vi "Teleop.vi"(10 "Match Info":T2={"Autonomous Elapsed Seconds"=0.0, "TeleOp Elapsed Seconds"=0.0, "Disabled Elapsed Seconds"=0.0, "Visited Autonomous"=FALSE, "Visited TeleOp"=FALSE, "Visited Disabled"=FALSE, "Autonomous Settings"={"Autonomous Style"=enum."Independent", "VI Refnum"=refnum}}, 11 "Call Context":T3) -> ()   [LabVIEW 2015]
doc: "This VI is called for each TeleOp packet received from the DS where the robot is not disabled. It is often used to read from the joysticks and update I/O or to update setpoints for timed control loops. It should complete and return within 20 milliseconds or it may miss DS packets."
uses:
  <vilib>/Rock Robotics/WPI/DriverStation/WPI_DriverStationDerivedRobotMode.ctl
  <vilib>/Rock Robotics/WPI/DriverStation/WPI_DriverStationMatch Info.ctl
  <vilib>/Rock Robotics/WPI/CAN/TalonSRX/WPI_CANTalonSRX_GlobalStatus.ctl
  <vilib>/Rock Robotics/WPI/Utilities/WPI_GetSetVariantRefNum.vi
  <vilib>/Rock Robotics/Network Tables/NT Write Boolean Array.vi
  <vilib>/Rock Robotics/Network Tables/NT Write Numeric Array.vi
  <vilib>/Rock Robotics/Network Tables/NT Read Boolean.vi
  <vilib>/Rock Robotics/Network Tables/NT Read Number.vi
  Stage.vi
panel:
  out "Set Point":dbl
  out "Talon SRX Status":T1
  out "Waveform Chart":cluster{"Encoder Velocity":dbl, dbl}(graph)
  out "Encoder Velocity":dbl
  out "Mode":bool
  out "Pos":bool
  out "Arm":dbl
  out "Optic":bool
  out "B10":bool
  out "B9":bool
  out "B8":bool
  out "Shooter rpm":dbl
  out "hooks motor":dbl
  out "Winch":dbl
  out "Stage3Motor":dbl
  out "Drive":dbl=0.5
  out "Stage1Motor":dbl
  out "Stage":dbl
  out "B7":bool
  out "ALU":bool
  out "ALB":bool
  out "B6":bool
  out "B5":bool
  out "LT":bool
  out "LM":bool
  out "LB":bool
  out "B4":bool
  out "B3":bool
  out "B2":bool
  out "B1":bool
  out "B0":bool
  out "Full speed":bool=TRUE
  out "Sample Slider 0":dbl(slide) scale=0.0..5.0
  out "Sample Boolean 1":bool
  out "Sample Boolean 0":bool
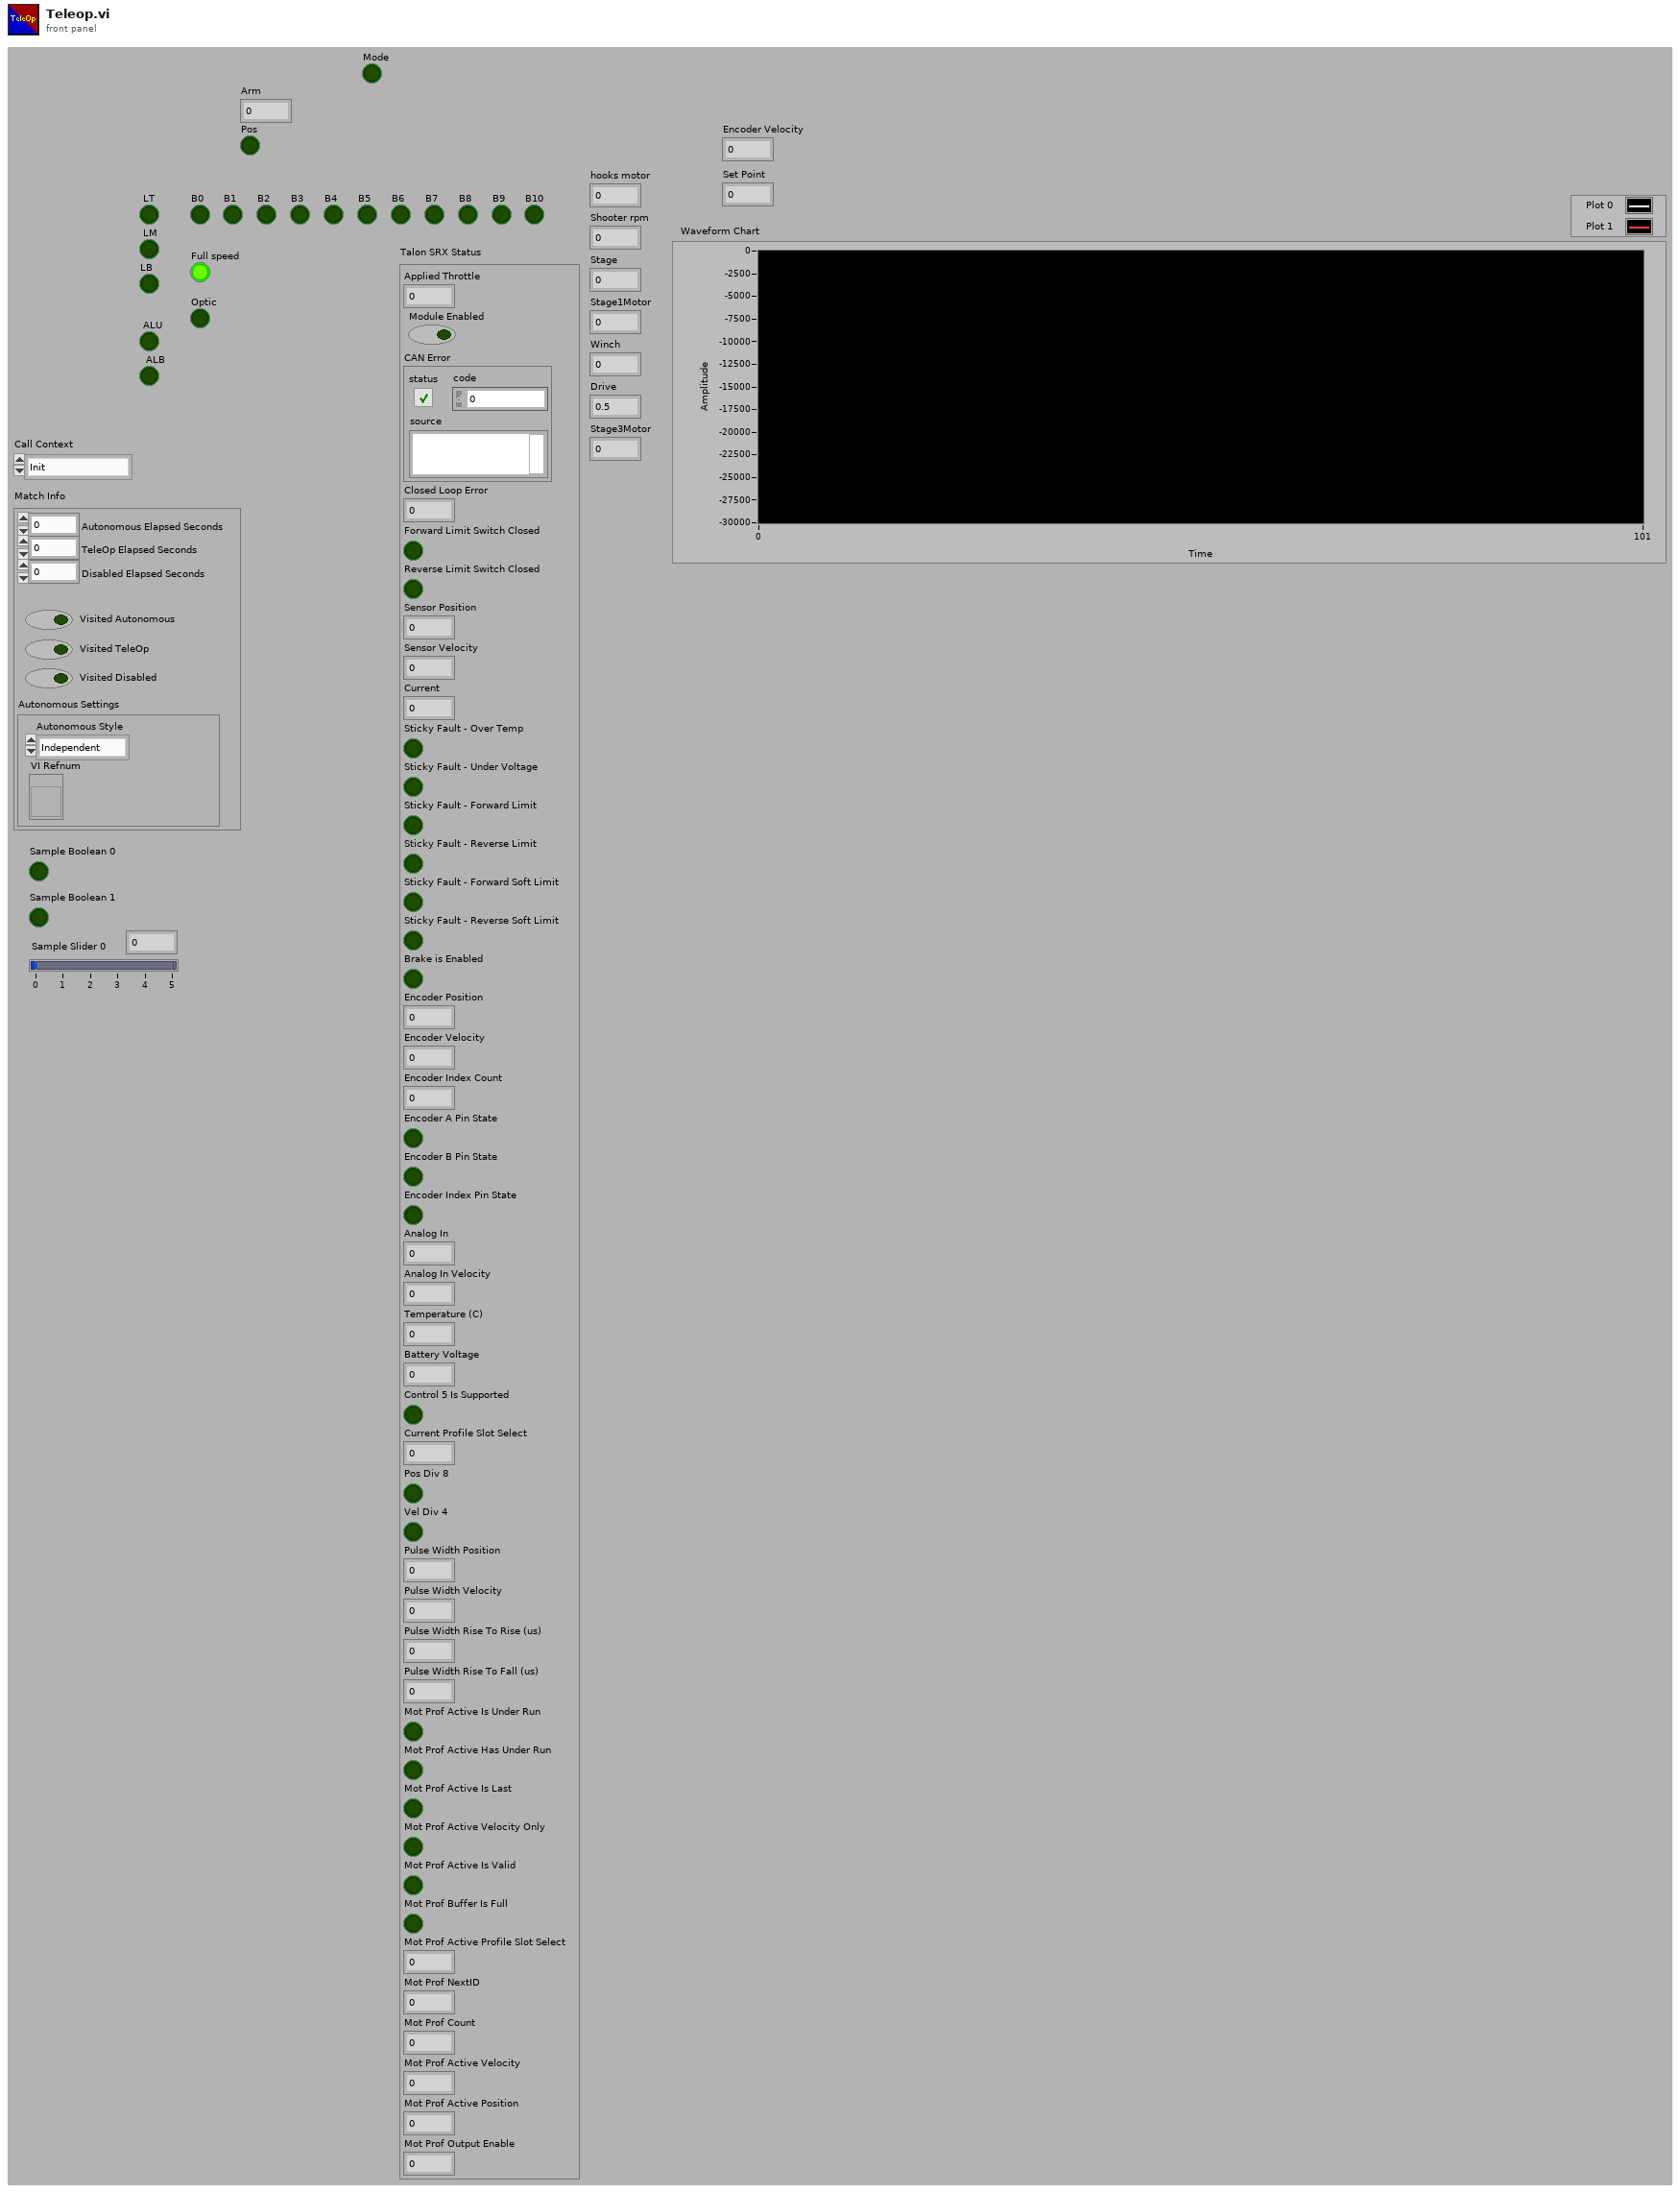
[diagram p1: front panel]
types:
  T1 = typedef "WPI_CANTalonSRX_GlobalStatus.ctl" = cluster{"Applied Throttle":dbl, "Module Enabled":bool, "CAN Error":errorcluster, "Closed Loop Error":dbl, "Forward Limit Switch Closed":bool, "Reverse Limit Switch Closed":bool, "Sensor Position":dbl, "Sensor Velocity":dbl, "Current":dbl, "Sticky Fault - Over Temp":bool, "Sticky Fault - Under Voltage":bool, "Sticky Fault - Forward Limit":bool, "Sticky Fault - Reverse Limit":bool, "Sticky Fault - Forward Soft Limit":bool, "Sticky Fault - Reverse Soft Limit":bool, "Brake is Enabled":bool, "Encoder Position":dbl, "Encoder Velocity":dbl, "Encoder Index Count":dbl, "Encoder A Pin State":bool, "Encoder B Pin State":bool, "Encoder Index Pin State":bool, "Analog In":dbl, "Analog In Velocity":dbl, "Temperature (C)":dbl, "Battery Voltage":dbl, "Control 5 Is Supported":bool, "Current Profile Slot Select":dbl, "Pos Div 8":bool, "Vel Div 4":bool, "Pulse Width Position":i32, "Pulse Width Velocity":i32, "Pulse Width Rise To Rise (us)":i32, "Pulse Width Rise To Fall (us)":i32, "Mot Prof Active Is Under Run":bool, "Mot Prof Active Has Under Run":bool, "Mot Prof Active Is Last":bool, "Mot Prof Active Velocity Only":bool, "Mot Prof Active Is Valid":bool, "Mot Prof Buffer Is Full":bool, "Mot Prof Active Profile Slot Select":i32, "Mot Prof NextID":i32, "Mot Prof Count":i32, "Mot Prof Active Velocity":dbl, "Mot Prof Active Position":dbl, "Mot Prof Output Enable":i32}
  T2 = typedef "WPI_DriverStationMatch Info.ctl" = cluster{"Autonomous Elapsed Seconds":dbl, "TeleOp Elapsed Seconds":dbl, "Disabled Elapsed Seconds":dbl, "Visited Autonomous":bool, "Visited TeleOp":bool, "Visited Disabled":bool, "Autonomous Settings":cluster{"Autonomous Style":enum16{"Iterative", "Independent"}, "VI Refnum":refnum<vi>}}
  T3 = typedef "WPI_DriverStationDerivedRobotMode.ctl" = enum16{"Init", "Execute", "Stop"}
  T4 = typedef "WPI_DigitalInputDevRef.ctl" = cluster{"DevStatus":errorcluster, "DIO Channel":T5}
  T5 = typedef "FPGA_DIOChannel.ctl" = enum8{"DIO 0", "DIO 1", "DIO 2", "DIO 3", "DIO 4", "DIO 5", "DIO 6", "DIO 7", "DIO 8", "DIO 9", "DIO MXP 0", "DIO MXP 1", "DIO MXP 2", "DIO MXP 3", "DIO MXP 4", "DIO MXP 5", "DIO MXP 6", "DIO MXP 7", "DIO MXP 8", "DIO MXP 9", "DIO MXP 10", "DIO MXP 11", "DIO MXP 12", "DIO MXP 13", "DIO MXP 14", "DIO MXP 15", "Invalid"}
  T6 = typedef "WPI_RobotDriveDevRef.ctl" = cluster{"DevStatus":errorcluster, "Motors[]":T7[], "Square Inputs":bool, "Max Output":dbl}
  T7 = typedef "WPI_MotorControlDeviceRef.ctl" = cluster{"DeviceStatus":errorcluster, "Type":T8, "PWM":cluster{"PWM Channel":T9, "DeadBand":T10}, "CAN":cluster{"Device Number":u8, "Control Mode":T11, "Semaphore":T12, "Max Vout":dbl, "TalonSRX Control Mode":T13}, "Invert":bool}
  T8 = typedef "WPI_MotorControlType.ctl" = enum16{"PWM", "CAN", "CANTalonSRX"}
  T9 = typedef "FPGA_DIOPWMChannel.ctl" = enum8{"PWM 0", "PWM 1", "PWM 2", "PWM 3", "PWM 4", "PWM 5", "PWM 6", "PWM 7", "PWM 8", "PWM 9", "PWM MXP 0", "PWM MXP 1", "PWM MXP 2", "PWM MXP 3", "PWM MXP 4", "PWM MXP 5", "PWM MXP 6", "PWM MXP 7", "PWM MXP 8", "PWM MXP 9", "Invalid"}
  T10 = typedef "WPI_PWMDeadband.ctl" = cluster{"Name":string, "maxPositivePwm":i32, "minPositivePwm":i32, "centerPwm":i32, "maxNegativePwm":i32, "minNegativePwm":i32, "angularRange":u16}
  T11 = typedef "WPI_CANJaguar_ControlMode.ctl" = enum8{"Percent VBus", "Current", "Speed", "Position", "Voltage"}
  T12 = typedef "Semaphore RefNum" = refnum<k1>
  T13 = typedef "WPI_CANTalonSRX_APIControlMode.ctl" = enum8{"Percent VBus", "Speed", "Position", "Slave", "Unchanged / Invalid", "Voltage Compensation", "Current", "Motion Profile"}
  T14 = typedef "WPI_JoystickDevRef.ctl" = cluster{"Device":T15}
  T15 = typedef "WPI_JoystickDeviceEnum.ctl" = enum16{"USB 0", "USB 1", "USB 2", "USB 3", "USB 4", "USB 5"}
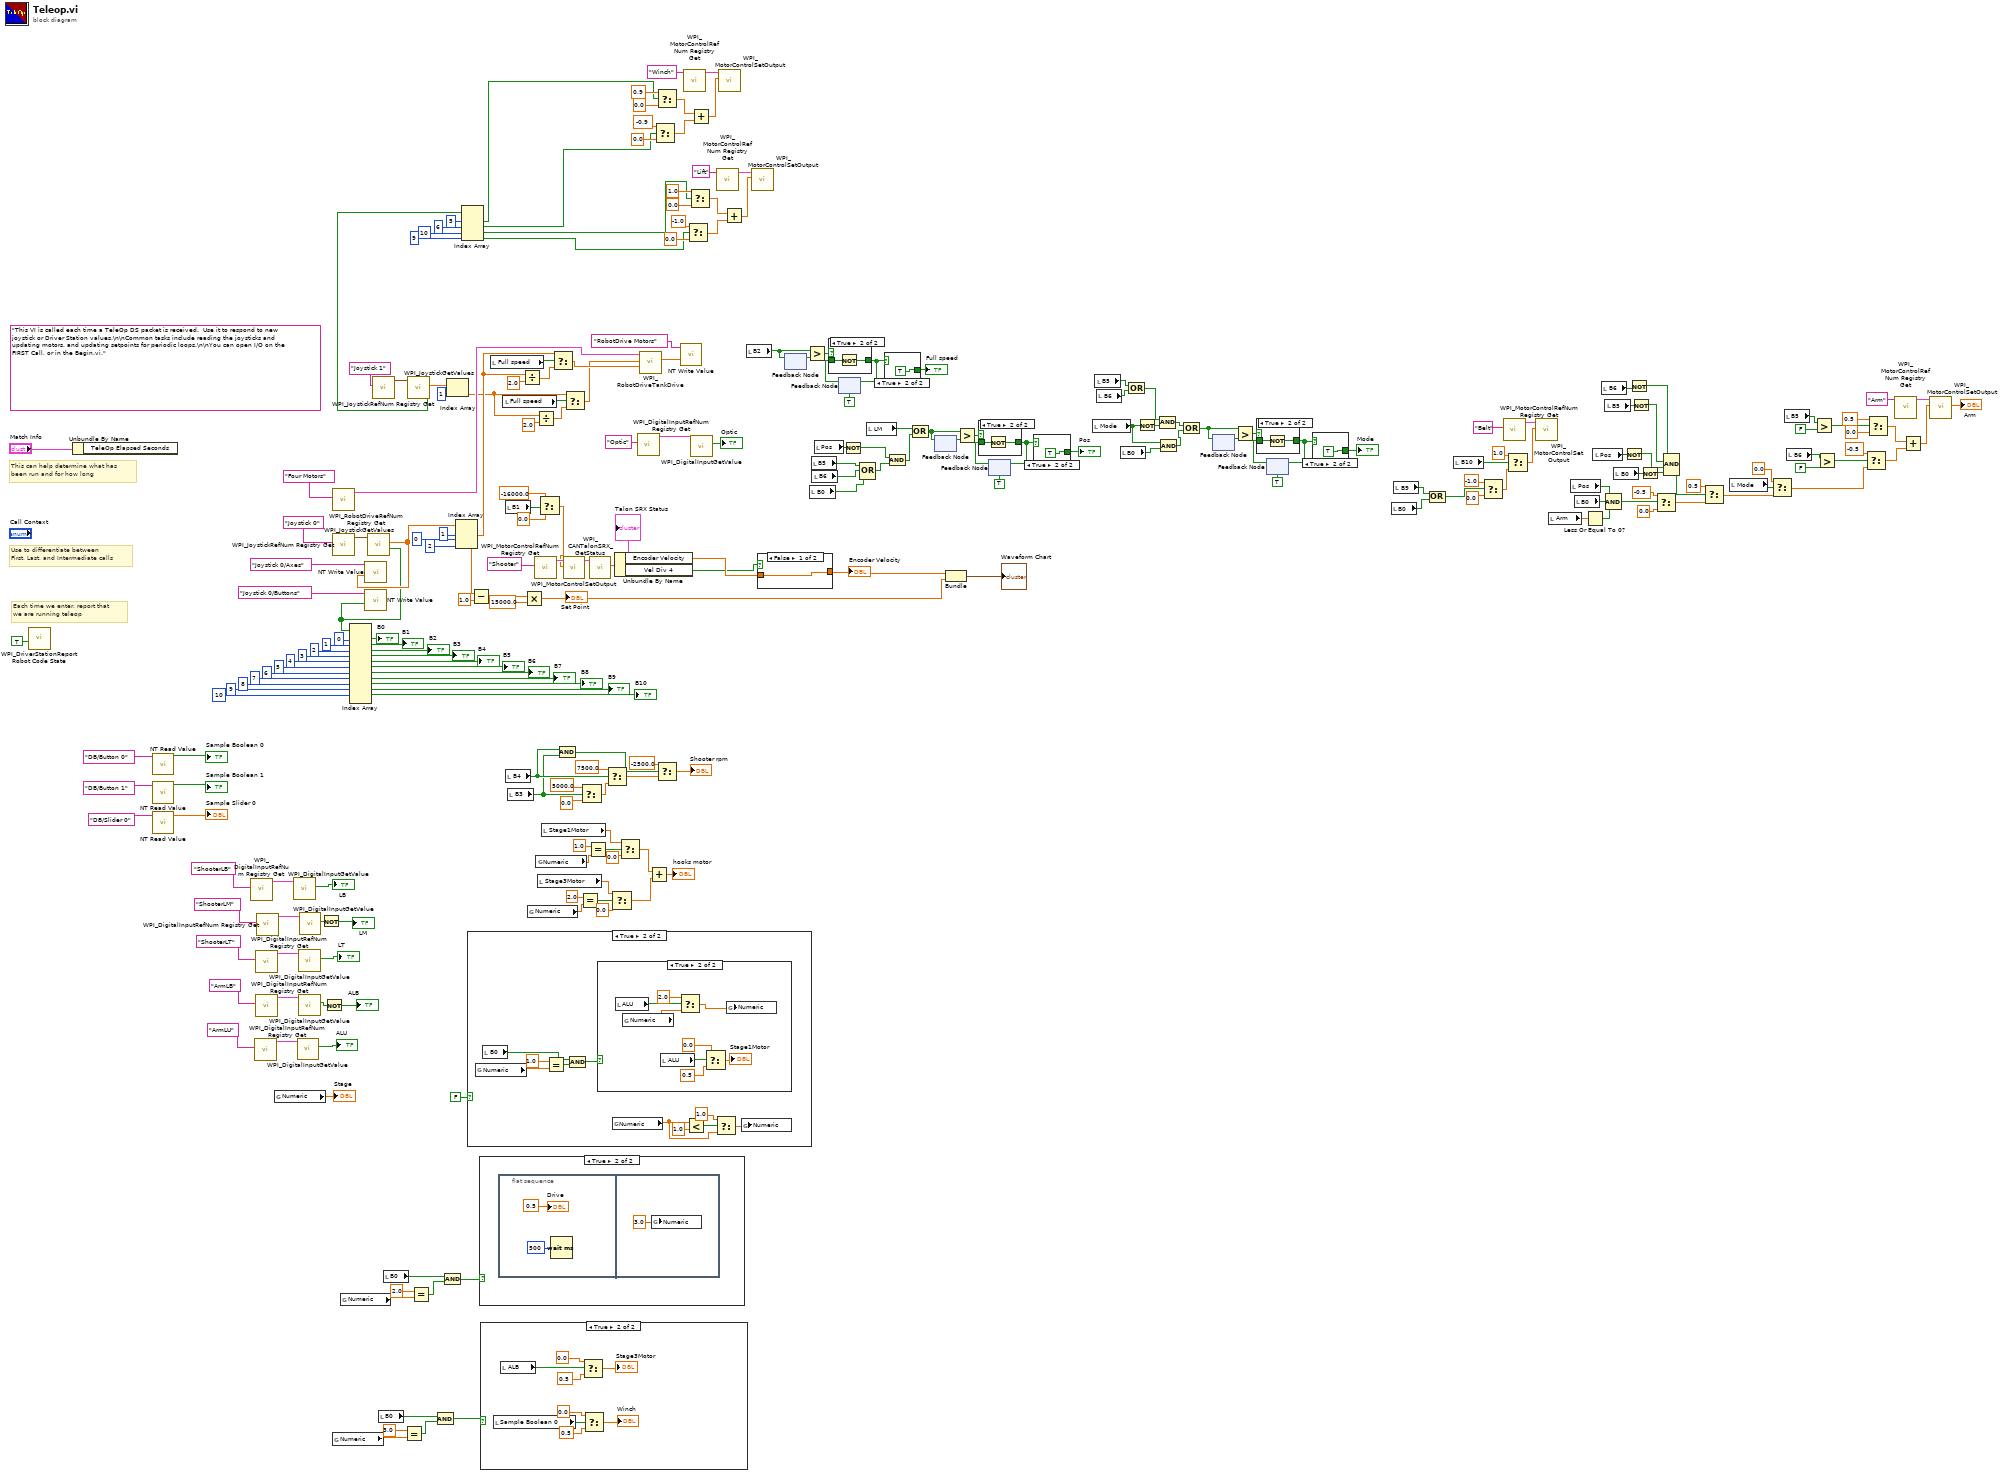
[diagram p0: block diagram]
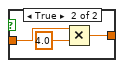
[diagram p2: hidden frame]
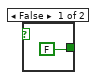
[diagram p3: hidden frame]
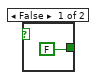
[diagram p5: hidden frame]
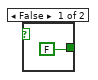
[diagram p11: hidden frame]
diagram:
  (unwired) "This VI is called each time a TeleOp DS packet is received.  Use it to respond to new joystick or Driver Station values.\n\nCommon tasks include reading the joysticks and updating motors, and updating setpoints for periodic loops.\n\nYou can open I/O on the FIRST Call, or in the Begin.vi."
  # "Each time we enter, report that\nwe are running teleop"
  # "Use to differentiate between\nFirst, Last, and Intermediate calls"
  # "This can help determine what has\nbeen run and for how long"
  n1 = call <vilib>:"WPI_DriverStationReport Robot Code State.vi"("TeleOp"=TRUE ("Autonomous")) -> ()  [unwired: 10 in, 1 out]
  n2 = Unbundle By Name("Match Info") -> ()  [unwired: 1 out]
  n3 = call-poly <vilib>:"NT Read Value.vi"("Name"="DB/Button 0" ("refnum name")) -> ("Boolean"=→"Sample Boolean 0":bool)  [unwired: 9 in, 1 out]
  n4 = call-poly <vilib>:"NT Read Value.vi"("Name"="DB/Button 1" ("refnum name")) -> ("Boolean"=→"Sample Boolean 1":bool)  [unwired: 9 in, 1 out]
  n5 = call-poly <vilib>:"NT Read Value.vi"("Name"="DB/Slider 0" ("refnum name")) -> ("Numeric"=→"Sample Slider 0":dbl)  [unwired: 9 in, 1 out]
  n6 = call <vilib>:"WPI_DigitalInputRefNum Registry Get.vi"("refnum name"="ShooterLB") -> ("DigitalInputDevRef"=w188:T4)  [unwired: 9 in, 1 out]
  n7 = call <vilib>:"WPI_DigitalInputRefNum Registry Get.vi"("refnum name"="ArmLU") -> ("DigitalInputDevRef"=w163:T4)  [unwired: 9 in, 1 out]
  n8 = call <vilib>:"WPI_DigitalInputRefNum Registry Get.vi"("refnum name"="ShooterLT") -> ("DigitalInputDevRef"=w183:T4)  [unwired: 9 in, 1 out]
  n9 = call <vilib>:"WPI_DigitalInputRefNum Registry Get.vi"("refnum name"="ArmLB") -> ("DigitalInputDevRef"=w164:T4)  [unwired: 9 in, 1 out]
  n10 = call <vilib>:"WPI_DigitalInputRefNum Registry Get.vi"("refnum name"="ShooterLM") -> ("DigitalInputDevRef"=w184:T4)  [unwired: 9 in, 1 out]
  n11 = global read "Stage.vi" "Numeric"() -> (→"Stage":dbl)
  n12 = call <vilib>:"WPI_DigitalInputGetValue.vi"("DigitalInputDevRef"=w188) -> ("Value"=→"LB":bool)  [unwired: 8 in, 2 out]
  n13 = call <vilib>:"WPI_DigitalInputGetValue.vi"("DigitalInputDevRef"=w163) -> ("Value"=→"ALU":bool)  [unwired: 8 in, 2 out]
  n14 = call <vilib>:"WPI_DigitalInputGetValue.vi"("DigitalInputDevRef"=w183) -> ("Value"=→"LT":bool)  [unwired: 8 in, 2 out]
  n15 = call <vilib>:"WPI_DigitalInputGetValue.vi"("DigitalInputDevRef"=w164) -> ("Value"=w20:bool)  [unwired: 8 in, 2 out]
  n16 = call <vilib>:"WPI_DigitalInputGetValue.vi"("DigitalInputDevRef"=w184) -> ("Value"=w83:bool)  [unwired: 8 in, 2 out]
  n17 = Not(x=w83) -> (.not. x?=→"LM":bool)
  n18 = Not(x=w20) -> (.not. x?=→"ALB":bool)
  n19 = call <vilib>:"WPI_RobotDriveRefNum Registry Get.vi"("refnum name"="Four Motors") -> ("RobotDriveDevRef"=w239:T6)  [unwired: 1 in, 9 out]
  n20 = call <vilib>:"WPI_JoystickRefNum Registry Get.vi"("refnum name"="Joystick 0") -> ("JoystickDevRef"=w237:T14)  [unwired: 1 in, 9 out]
  n21 = global read "Stage.vi" "Numeric"() -> (w150:dbl)
  n22 = global read "Stage.vi" "Numeric"() -> (w154:dbl)
  n23 = call <vilib>:"WPI_JoystickGetValues.vi"("JoystickDevRef"=w237) -> ("Buttons"=w224:bool[], "Axes"=w234:dbl[])  [unwired: 6 in, 3 out]
  n24 = Index Array(array=w224, index #1=0 ("index"), index #2=1 ("index"), index #3=2 ("index"), index #4=3 ("index"), index #5=4 ("index"), index #6=5 ("index"), index #7=6 ("index"), index #8=7 ("index"), index #9=8 ("index"), index #10=9 ("index"), index #11=10 ("index")) -> (element #1=→"B0":bool, element #2=→"B1":bool, element #3=→"B2":bool, element #4=→"B3":bool, element #5=→"B4":bool, element #6=→"B5":bool, element #7=→"B6":bool, element #8=→"B7":bool, element #9=→"B8":bool, element #10=→"B9":bool, element #11=→"B10":bool)  [unwired: 1 in, 1 out]
  n25 = call-poly <vilib>:"NT Write Value.vi"("Numeric Array"=w234, "Name"="Joystick 0/Axes") -> ()  [unwired: 9 in, 1 out]
  n26 = call-poly <vilib>:"NT Write Value.vi"("Boolean Array"=w224, "Name"="Joystick 0/Buttons") -> ()  [unwired: 9 in, 1 out]
  n27 = call <vilib>:"WPI_JoystickRefNum Registry Get.vi"("refnum name"="Joystick 1") -> ("JoystickDevRef"=w114:T14)  [unwired: 1 in, 9 out]
  n28 = local read "B0"() -> (w146:bool)
  n29 = local read "B0"() -> (w155:bool)
  n30 = Equal?(x=3.0, y=w150) -> (x = y?=w148:bool)
  n31 = call <vilib>:"WPI_JoystickGetValues.vi"("JoystickDevRef"=w114) -> ("Buttons"=w59:bool[], "Axes"=w113:dbl[])  [unwired: 6 in, 3 out]
  n32 = Equal?(x=2.0, y=w154) -> (x = y?=w152:bool)
  n33 = Compound Arithmetic op=AND(w146, w148) -> (w147:bool)
  n34 = Compound Arithmetic op=AND(w155, w152) -> (w151:bool)
  n35 = Index Array(array=w113, index=1) -> (element=w112:dbl)
  n36 = Index Array(array=w234, index #1=1 ("index"), index #2=0 ("index"), index #3=2 ("index")) -> (element #1=w216:dbl, element #3=w12:dbl)  [unwired: 1 out]
  n37 = Index Array(array=w59, index #1=5 ("index"), index #2=6 ("index"), index #3=10 ("index"), index #4=9 ("index")) -> (element #1=w4:bool, element #2=w3:bool, element #3=w2:bool, element #4=w1:bool)
  n38 = case shown="True" FALSE {
    frame False {
    }
    frame True {
      n39 = global read "Stage.vi" "Numeric"() -> (w246:dbl)
      n40 = local read "B0"() -> (w243:bool)
      n41 = Equal?(x=1.0, y=w246) -> (x = y?=w244:bool)
      n42 = Compound Arithmetic op=AND(w243, w244) -> (w242:bool)
      n43 = case shown="True" w242 {
        frame False {
        }
        frame True {
          n44 = local read "ALU"() -> (w255:bool)
          n45 = global read "Stage.vi" "Numeric"() -> (w253:dbl)
          n46 = local read "ALU"() -> (w259:bool)
          n47 = Select(t=2.0, s=w255, f=w253) -> (s? t:f=w254:dbl)
          n48 = Select(t=0.0, s=w259, f=0.5) -> (s? t:f=→"Stage1Motor":dbl)
          n49 = global write "Stage.vi" "Numeric"(w254) -> ()
        }
      }
      n50 = global read "Stage.vi" "Numeric"() -> (w248:dbl)
      n51 = Less?(x=w248, y=1.0) -> (x < y?=w250:bool)
      n52 = Select(t=1.0, s=w250, f=w248) -> (s? t:f=w247:dbl)
      n53 = global write "Stage.vi" "Numeric"(w247) -> ()
    }
  }
  n54 = Subtract(x=w12, y=1.0) -> (x-y=w14:dbl)
  n55 = case shown="True" w151 {
    frame False {
    }
    frame True {
      n56 = flat-sequence {
        frame #0 {
          n57 = Wait (ms)(milliseconds to wait=u32 500) -> ()  [unwired: 1 out]
          "Drive" <- 0.5
        }
        frame #1 {
          n58 = global write "Stage.vi" "Numeric"(3.0 ("Numeric")) -> ()
        }
      }
    }
  }
  n59 = case shown="True" w147 {
    frame False {
    }
    frame True {
      n60 = local read "Sample Boolean 0"() -> (w263:bool)
      n61 = local read "ALB"() -> (w268:bool)
      n62 = Select(t=0.0, s=w268, f=0.5) -> (s? t:f=→"Stage3Motor":dbl)
      n63 = Select(t=0.0, s=w263, f=0.5) -> (s? t:f=→"Winch":dbl)
    }
  }
  n64 = local read "Full speed"() -> (w212:bool)
  n65 = local read "Full speed"() -> (w206:bool)
  n66 = local read "B1"() -> (w9:bool)
  n67 = local read "B4"() -> (w195:bool)
  n68 = local read "B3"() -> (w194:bool)
  n69 = Divide(x=w216, y=2.0) -> (x/y=w215:dbl)
  n70 = Multiply(x=w14, y=15000.0) -> (x*y=w7:dbl)
  "Set Point" <- w7
  n71 = global read "Stage.vi" "Numeric"() -> (w143:dbl)
  n72 = call <vilib>:"WPI_MotorControlRefNum Registry Get.vi"("refnum name"="Shooter") -> ("MotorControlDevRef"=w189:T7)  [unwired: 9 in, 1 out]
  n73 = Divide(x=w112, y=2.0) -> (x/y=w204:dbl)
  n74 = global read "Stage.vi" "Numeric"() -> (w145:dbl)
  n75 = local read "Stage3Motor"() -> (w137:dbl)
  n76 = Select(t=-16000.0, s=w9, f=0.0) -> (s? t:f=w8:dbl)
  n77 = local read "Stage1Motor"() -> (w139:dbl)
  n78 = Select(t=w216, s=w212, f=w215) -> (s? t:f=w107:dbl)
  n79 = And(x=w195, y=w194) -> (x .and. y?=w193:bool)
  n80 = call <vilib>:"WPI_MotorControlSetOutput.vi"("Output"=w8, "MotorControlDevRef"=w189) -> ("MotorControlDevRef"=w19:T7)  [unwired: 7 in, 2 out]
  n81 = Select(t=w112, s=w206, f=w204) -> (s? t:f=w106:dbl)
  n82 = Equal?(x=2.0, y=w143) -> (x = y?=w138:bool)
  n83 = Select(t=5000.0, s=w194, f=0.0) -> (s? t:f=w198:dbl)
  n84 = Equal?(x=1.0, y=w145) -> (x = y?=w141:bool)
  n85 = call <vilib>:"WPI_CANTalonSRX_GetStatus.vi"("CAN Talon SRX Ref"=w19) -> ("Talon SRX Status"=w18:T1)  [unwired: 8 in, 2 out]
  "Talon SRX Status" <- w18
  n86 = Select(t=7500.0, s=w195, f=w198) -> (s? t:f=w192:dbl)
  n87 = Select(t=w137, s=w138, f=0.0) -> (s? t:f=w134:dbl)
  n88 = Unbundle By Name(w18) -> ("Encoder Velocity"=w17:dbl, "Vel Div 4"=w16:bool)
  n89 = Select(t=w139, s=w141, f=0.0) -> (s? t:f=w135:dbl)
  n90 = call <vilib>:"WPI_DigitalInputRefNum Registry Get.vi"("refnum name"="Optic") -> ("DigitalInputDevRef"=w110:T4)  [unwired: 9 in, 1 out]
  n91 = call <vilib>:"WPI_RobotDriveTankDrive.vi"("Right axis value"=w107, "Left axis value"=w106, "RobotDriveDevRef"=w239) -> ("Motor Values"=w232:dbl[])  [unwired: 6 in, 2 out]
  n92 = Add(x=w135, y=w134) -> (x+y=→"hooks motor":dbl)
  n93 = Select(t=-0.9, s=w3, f=0.0) -> (s? t:f=w50:dbl)
  n94 = Select(t=0.9, s=w4, f=0.0) -> (s? t:f=w49:dbl)
  n95 = Select(t=-2500.0, s=w193, f=w192) -> (s? t:f=→"Shooter rpm":dbl)
  n96 = call-poly <vilib>:"NT Write Value.vi"("Numeric Array"=w232, "Name"="RobotDrive Motors") -> ()  [unwired: 9 in, 1 out]
  n97 = call <vilib>:"WPI_MotorControlRefNum Registry Get.vi"("refnum name"="Winch") -> ("MotorControlDevRef"=w55:T7)  [unwired: 9 in, 1 out]
  n98 = Select(t=-1.0, s=w1, f=0.0) -> (s? t:f=w64:dbl)
  n99 = Select(t=1.0, s=w2, f=0.0) -> (s? t:f=w63:dbl)
  n100 = Add(x=w49, y=w50) -> (x+y=w47:dbl)
  n101 = call <vilib>:"WPI_DigitalInputGetValue.vi"("DigitalInputDevRef"=w110) -> ("Value"=→"Optic":bool)  [unwired: 8 in, 2 out]
  n102 = call <vilib>:"WPI_MotorControlRefNum Registry Get.vi"("refnum name"="Lift") -> ("MotorControlDevRef"=w69:T7)  [unwired: 9 in, 1 out]
  n103 = call <vilib>:"WPI_MotorControlSetOutput.vi"("Output"=w47, "MotorControlDevRef"=w55) -> ()  [unwired: 7 in, 3 out]
  n104 = Add(x=w63, y=w64) -> (x+y=w61:dbl)
  n105 = local read "B2"() -> (w208:bool)
  n106 = call <vilib>:"WPI_MotorControlSetOutput.vi"("Output"=w61, "MotorControlDevRef"=w69) -> ()  [unwired: 7 in, 3 out]
  n107 = case shown="False" w16 {
    tunnel: [w271 w274] -> w11
    tunnel: w17 -> [w271 w272]
    frame False {
    }
    frame True {
      n108 = Multiply(x=w272, y=4.0) -> (x*y=w274:dbl)
    }
  }
  "Encoder Velocity" <- w11
  n109 = feedback-in #1(w208) -> ()
  n110 = feedback #1() -> (w207:bool)  [unwired: 1 in]
  n111 = Greater?(x=w208, y=w207) -> (0:w220:bool)
  n112 = local read "B0"() -> (w76:bool)
  n113 = local read "B5"() -> (w78:bool)
  n114 = local read "B6"() -> (w77:bool)
  n115 = local read "Pos"() -> (w80:bool)
  n116 = feedback #2(TRUE) -> (w219:bool)
  n117 = case shown="True" w220 {
    tunnel: [w275 w277] -> w218
    tunnel: w219 -> [w275 w276]
    frame False {
    }
    frame True {
      n118 = Not(x=w276) -> (.not. x?=w277:bool)
    }
  }
  n119 = feedback-in #2(w218) -> ()
  n120 = Not(x=w80) -> (.not. x?=w74:bool)
  n121 = Compound Arithmetic op=OR(w78, w77, w76) -> (w75:bool)
  n122 = local read "LM"() -> (w42:bool)
  n123 = case shown="True" w218 {
    tunnel: [FALSE TRUE] -> w214
    frame False {
    }
    frame True {
    }
  }
  "Full speed" <- w214
  n124 = Compound Arithmetic op=AND(w74, w75) -> (w79:bool)
  n125 = Compound Arithmetic op=OR(w42, w79) -> (w81:bool)
  n126 = feedback #3() -> (w92:bool)  [unwired: 1 in]
  n127 = feedback-in #3(w81) -> ()
  n128 = Bundle("Encoder Velocity"=w11, w7) -> (→"Waveform Chart":cluster{"Encoder Velocity":dbl, dbl})  [unwired: 1 in]
  n129 = Greater?(x=w81, y=w92) -> (0:w96:bool)
  n130 = feedback #4(TRUE) -> (w95:bool)
  n131 = case shown="True" w96 {
    tunnel: [w280 w282] -> w94
    tunnel: w95 -> [w280 w281]
    frame False {
    }
    frame True {
      n132 = Not(x=w281) -> (.not. x?=w282:bool)
    }
  }
  n133 = feedback-in #4(w94) -> ()
  n134 = case shown="True" w94 {
    tunnel: [FALSE TRUE] -> w91
    frame False {
    }
    frame True {
    }
  }
  "Pos" <- w91
  n135 = local read "Mode"() -> (w30:bool)
  n136 = local read "B5"() -> (w35:bool)
  n137 = local read "B6"() -> (w34:bool)
  n138 = local read "B0"() -> (w29:bool)
  n139 = Compound Arithmetic op=OR(w35, w34) -> (w33:bool)
  n140 = Not(x=w30) -> (.not. x?=w32:bool)
  n141 = Compound Arithmetic op=AND(w33, w32) -> (w31:bool)
  n142 = Compound Arithmetic op=AND(w30, w29) -> (w28:bool)
  n143 = Compound Arithmetic op=OR(w31, w28) -> (w27:bool)
  n144 = feedback #5() -> (w37:bool)  [unwired: 1 in]
  n145 = feedback-in #5(w27) -> ()
  n146 = Greater?(x=w27, y=w37) -> (0:w41:bool)
  n147 = feedback #6(TRUE) -> (w40:bool)
  n148 = case shown="True" w41 {
    tunnel: [w285 w287] -> w39
    tunnel: w40 -> [w285 w286]
    frame False {
    }
    frame True {
      n149 = Not(x=w286) -> (.not. x?=w287:bool)
    }
  }
  n150 = feedback-in #6(w39) -> ()
  n151 = case shown="True" w39 {
    tunnel: [FALSE TRUE] -> w36
    frame False {
    }
    frame True {
    }
  }
  "Mode" <- w36
  n152 = local read "B0"() -> (w71:bool)
  n153 = local read "B9"() -> (w73:bool)
  n154 = Compound Arithmetic op=OR(w73, w71) -> (w72:bool)
  n155 = local read "B10"() -> (w119:bool)
  n156 = Select(t=-1.0, s=w72, f=0.0) -> (s? t:f=w121:dbl)
  n157 = call <vilib>:"WPI_MotorControlRefNum Registry Get.vi"("refnum name"="Belt") -> ("MotorControlDevRef"=w156:T7)  [unwired: 9 in, 1 out]
  n158 = Select(t=1.0, s=w119, f=w121) -> (s? t:f=w120:dbl)
  n159 = call <vilib>:"WPI_MotorControlSetOutput.vi"("Output"=w120, "MotorControlDevRef"=w156) -> ()  [unwired: 7 in, 3 out]
  n160 = local read "Arm"() -> (w103:dbl)
  n161 = local read "Pos"() -> (w90:bool)
  n162 = local read "B0"() -> (w104:bool)
  n163 = Less Or Equal To 0?(x=w103) -> (x <= 0?=w102:bool)
  n164 = local read "Pos"() -> (w89:bool)
  n165 = local read "B6"() -> (w46:bool)
  n166 = local read "B5"() -> (w45:bool)
  n167 = Compound Arithmetic op=AND(w90, w104, w102) -> (w101:bool)
  n168 = local read "B0"() -> (w88:bool)
  n169 = Not(x=w89) -> (.not. x?=w87:bool)
  n170 = Not(x=w46) -> (.not. x?=w44:bool)
  n171 = Not(x=w45) -> (.not. x?=w43:bool)
  n172 = Not(x=w88) -> (.not. x?=w86:bool)
  n173 = Select(t=-0.5, s=w101, f=0.0) -> (s? t:f=w98:dbl)
  n174 = Compound Arithmetic op=AND(w44, w43, w87, w86) -> (w85:bool)
  n175 = Select(t=0.5, s=w85, f=w98) -> (s? t:f=w26:dbl)
  n176 = local read "Mode"() -> (w25:bool)
  n177 = Select(t=0.0, s=w25, f=w26) -> (s? t:f=w23:dbl)
  n178 = local read "B5"() -> (w174:bool)
  n179 = local read "B6"() -> (w170:bool)
  n180 = Greater?(x=w174, y=FALSE) -> (0:w173:bool)
  n181 = Greater?(x=w170, y=FALSE) -> (0:w169:bool)
  n182 = Select(t=-0.5, s=w169, f=w23) -> (s? t:f=w167:dbl)
  n183 = Select(t=0.5, s=w173, f=0.0) -> (s? t:f=w166:dbl)
  n184 = call <vilib>:"WPI_MotorControlRefNum Registry Get.vi"("refnum name"="Arm") -> ("MotorControlDevRef"=w176:T7)  [unwired: 9 in, 1 out]
  n185 = Add(x=w166, y=w167) -> (x+y=w70:dbl)
  n186 = call <vilib>:"WPI_MotorControlSetOutput.vi"("Output"=w70, "MotorControlDevRef"=w176) -> ("Motor Output"=→"Arm":dbl)  [unwired: 7 in, 2 out]
